vi "Time CNV.vi"(11 "时间标识":timestamp) -> (3 "字符串":string)   [LabVIEW 2016, in "DGUS.lvlib" / "DGUS.lvclass"]
uses:
  DGUS.lvclass
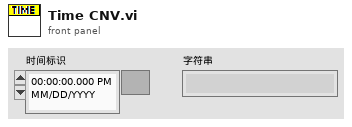
[diagram p1: front panel]
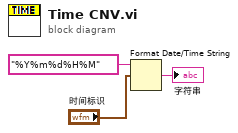
[diagram p0: block diagram]
diagram:
  n1 = Format Date/Time String(time format string (%c)="%Y%m%d%H%M" ("时间格式字符串(%c)"), seconds (now)="时间标识") -> (date/time string=→"字符串":string)  [unwired: 1 in]
